vi "Flush TCP Buffer.vi"(0 "CART TCP Connection In":refnum<k5>, 11 "error in (no error)":errorcluster) -> (4 "CART TCP Connection Out":refnum<k5>, 15 "error out":errorcluster)   [LabVIEW 2012]
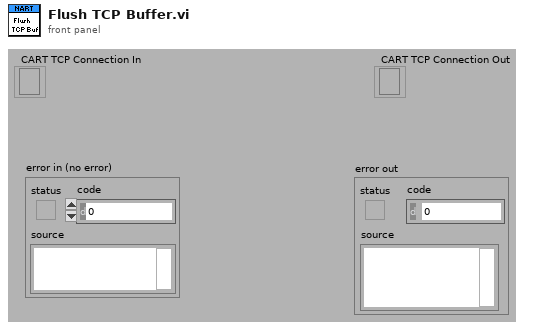
[diagram p1: front panel]
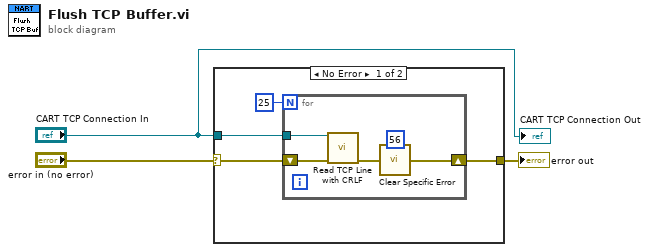
[diagram p0: block diagram]
diagram:
  n1 = case shown="No Error" "error in (no error)" {
    selector: "error in (no error)" -> [w5 w13]
    tunnel: "CART TCP Connection In" -> [w6 _]
    tunnel: [w4 w13] -> w1
    frame No Error {
      n2 = for {
        N: 25 -> [_]
        tunnel: w6 -> [w12]
        shift-right: [w8] -> w4
        shift-left: w5 -> [w11]
        n3 = call "Read TCP Line with CRLF.vi"("TCP Connection In"=w12, "error in"=w11) -> ("error out"=w9:errorcluster)  [unwired: 11 in, 2 out]
        n4 = call "Clear Specific Error.vi"("Specific Error Number (0: none)"=56, "error in"=w9) -> ("error out"=w8:errorcluster)  [unwired: 12 in, 1 out]
      }
    }
    frame Error {
    }
  }
  "error out" <- w1
  "CART TCP Connection Out" <- "CART TCP Connection In"
